vi "CTRE_Phoenix_CANcoder_GetSensorData.vi"(0 "CTRE_CANcoder_DeviceRef":T1, 11 "error in":errorcluster) -> (4 "CTRE_CANcoder_DeviceRef":T1, 6 "Position":dbl, 8 "Velocity":dbl, 10 "Absolute Position":dbl, 15 "error out":errorcluster)   [LabVIEW 2019]
doc: "Returns the sensor position and velocity of the CANcoder.\nThe units are determined by the coefficient and unit-string configuration parameters.\n\n<b>Position</b> default units are degrees.\n<b>Velocity</b> default units are degrees per second.\n<b>Absolute Position</b> default units are degrees. The absolute position may be unsigned (for example: [0,360) deg), or signed (for example: [-180,+180) deg). This is determined by a configuration. The default selection is unsigned."
uses:
  <vilib>/Rock Robotics/WPI/ThirdParty/Phoenix-LabVIEW/CANCoder/CTRE_Phoenix_CANcoder_DeviceRef.ctl
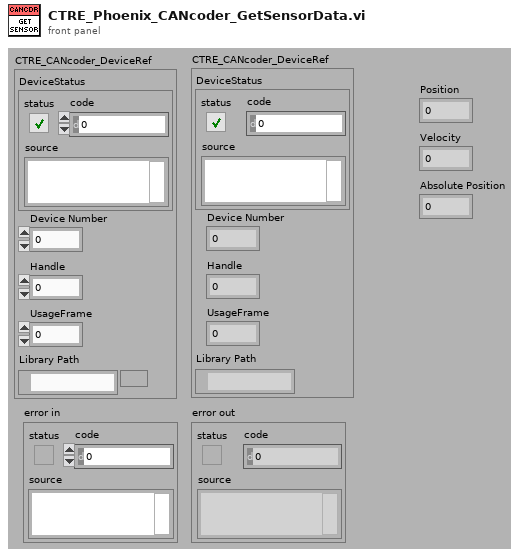
[diagram p1: front panel]
types:
  T1 = typedef "CTRE_Phoenix_CANcoder_DeviceRef.ctl" = cluster{"DeviceStatus":errorcluster, "Device Number":u8, "Handle":u64, "UsageFrame":u32, "Library Path":path}
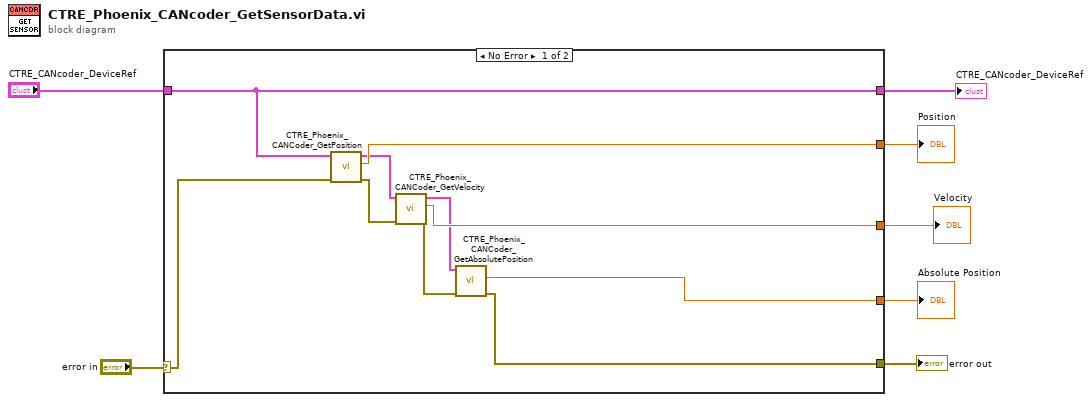
[diagram p0: block diagram]
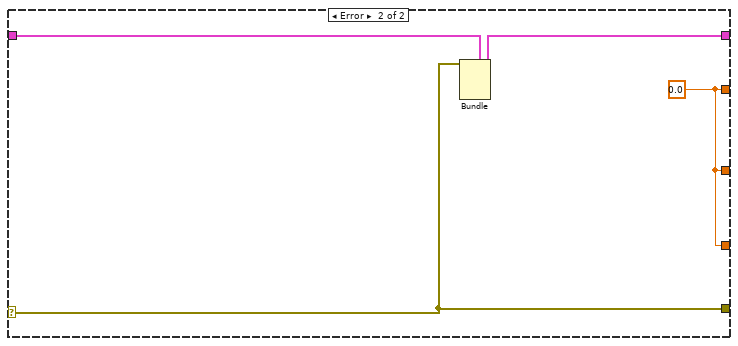
[diagram p2: hidden frame]
diagram:
  n1 = case shown="No Error" "error in" {
    selector: "error in" -> [w16 w20]
    tunnel: "CTRE_CANcoder_DeviceRef" -> [w17 w21]
    tunnel: [w8 w20] -> w7
    tunnel: [w17 w19] -> w2
    tunnel: [w15 w18] -> w5
    tunnel: [w12 w18] -> w4
    tunnel: [w11 w18] -> w1
    frame No Error {
      n2 = call <vilib>:"CTRE_Phoenix_CANCoder_GetPosition.vi"("error in"=w16, "CTRE_CANcoder_DeviceRef"=w17) -> ("error out"=w14:errorcluster, "Position (Scaled)"=w15:dbl, "CTRE_CANcoder_DeviceRef"=w13:T1)  [unwired: 7 in]
      n3 = call <vilib>:"CTRE_Phoenix_CANCoder_GetVelocity.vi"("error in"=w14, "CTRE_CANcoder_DeviceRef"=w13) -> ("error out"=w10:errorcluster, "Velocity"=w12:dbl, "CTRE_CANcoder_DeviceRef"=w9:T1)  [unwired: 7 in]
      n4 = call <vilib>:"CTRE_Phoenix_CANCoder_GetAbsolutePosition.vi"("error in"=w10, "CTRE_CANcoder_DeviceRef"=w9) -> ("error out"=w8:errorcluster, "Absolute Position"=w11:dbl)  [unwired: 7 in, 1 out]
    }
    frame Error {
      w18 = 0.0 ("Position (Raw Sensor Units)")
      n5 = Bundle(cluster=w21, "DeviceStatus"=w20) -> (w19:T1)  [unwired: 4 in]
    }
  }
  "error out" <- w7
  "Position" <- w5
  "Velocity" <- w4
  "CTRE_CANcoder_DeviceRef" <- w2
  "Absolute Position" <- w1
